vi "Init Serial.vi"(2 "VISA resource name":refnum<visa-resource-name>="COM9", 3 "baud rate":u32=115200) -> (0 "error out":errorcluster, 1 "VISA resource name out":refnum<visa-resource-name>)   [LabVIEW 2013]
uses:
  <vilib>/Instr/_visa.llb/VISA Configure Serial Port (Instr).vi
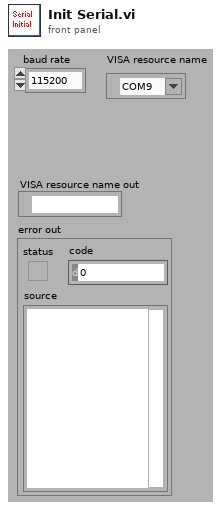
[diagram p1: front panel]
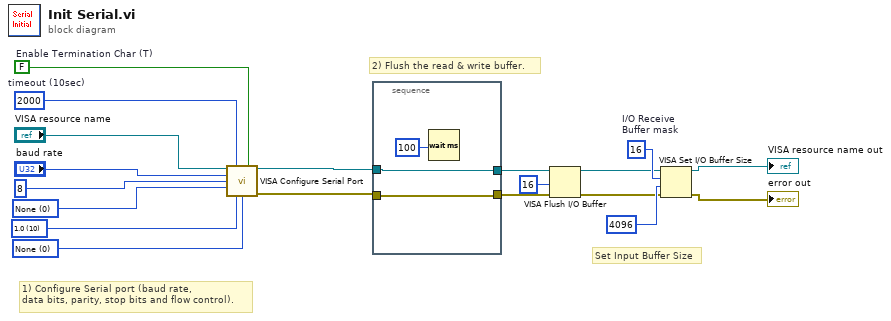
[diagram p0: block diagram]
diagram:
  w11 = u16 16  # I/O Receive Buffer mask
  w18 = u16 0 items=["None"=0, "XON/XOFF"=1, "RTS/CTS"=2, "DTR/DSR"=4] ("flow control")
  w17 = u16 10 items=["1.0"=10, "1.5"=15, "2.0"=20] ("stop bits")
  w15 = u16 0 items=["None", "Odd", "Even", "Mark", "Space"] ("parity")
  w12 = FALSE  # Enable Termination Char (T)
  w16 = u32 2000  # timeout (10sec)
  # "Set Input Buffer Size"
  # "2) Flush the read & write buffer."
  # "1) Configure Serial port (baud rate,\ndata bits, parity, stop bits and flow control)."
  n1 = call-poly "VISA Configure Serial Port"("VISA resource name"="VISA resource name", "timeout (10sec)"=w16, "Enable Termination\nChar (T)"=w12, "baud rate (9600)"="baud rate", "data bits (8)"=u16 8 ("data bits"), "parity (0:none)"=w15, "stop bits (10: 1 bit)"=w17, "flow control (0:none)"=w18) -> ("VISA resource name out"=w2:refnum<visa-resource-name>, "error out"=w1:errorcluster)  [unwired: 1 in, 5 out]
  n2 = stacked-sequence {
    tunnel: [w21] -> w5
    tunnel: [w22] -> w6
    tunnel: w2 -> [w22]
    tunnel: w1 -> [w21]
    frame #0 {
      n3 = Wait (ms)(milliseconds to wait=100) -> ()  [unwired: 1 out]
    }
  }
  n4 = VISA Flush I/O Buffer(VISA resource name=w6, mask (16)=u16 16, error in (no error)=w5) -> (VISA resource name out=w8:refnum<visa-resource-name>, error out=w7:errorcluster)
  n5 = VISA Set I/O Buffer Size(VISA resource name=w8, mask (16)=w11, size (4096)=u32 4096 ("Input\nbuffer size"), error in (no error)=w7) -> (VISA resource name out=→"VISA resource name out":refnum<visa-resource-name>, error out=→"error out":errorcluster)
